vi "ForceSettingsQuantized.vi"(9 "Function":i32) -> (1 "k":dbl format="%#_13g", 2 "Setpoint":dbl format="%#_13g")   [LabVIEW 2023]
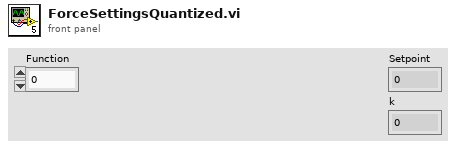
[diagram p1: front panel]
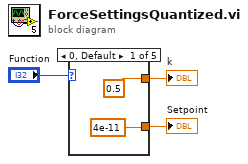
[diagram p0: block diagram]
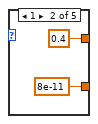
[diagram p2: hidden frame]
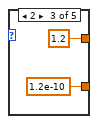
[diagram p3: hidden frame]
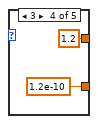
[diagram p4: hidden frame]
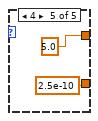
[diagram p5: hidden frame]
diagram:
  n1 = case shown="0, Default" "Function" {
    tunnel: [0.5 0.4 1.2 1.2 5.0] -> w2
    tunnel: [4e-11 8e-11 1.2e-10 1.2e-10 2.5e-10] -> w1
    frame 0, Default {
    }
    frame 1 {
    }
    frame 2 {
    }
    frame 3 {
    }
    frame 4 {
    }
  }
  "Setpoint" <- w1
  "k" <- w2
